vi "AutoWfmToSpreadsheet_2017.vi"() -> ()   [LabVIEW 2017]
uses:
  <vilib>/Waveform/WDTFileIO.llb/Read Waveform from File.vi
  <vilib>/Waveform/WDTFileIO.llb/Export Waveforms To Spreadsheet File (1D).vi
  <vilib>/Waveform/WDTOps.llb/WDT Index Channel DBL.vi
panel:
  out "?":string
  out "Sinal adquirido":waveform(dbl)(graph)
  in  "?":bool
  in  "Escolher arquivo":i32
  out "Sinal de Referência":waveform(dbl)(graph)
  in  "V para Exportar/ F para Visualizar":bool
  out "result string":string
  in  "Local da pasta com arquivos wfm":path=path "C:/Users/lucas/Documents/GitHub/INT/Novo Ensaio US/NOVOS_SINAIS/sinais/wfm"
  out "element":string
  out "Numeric":i32
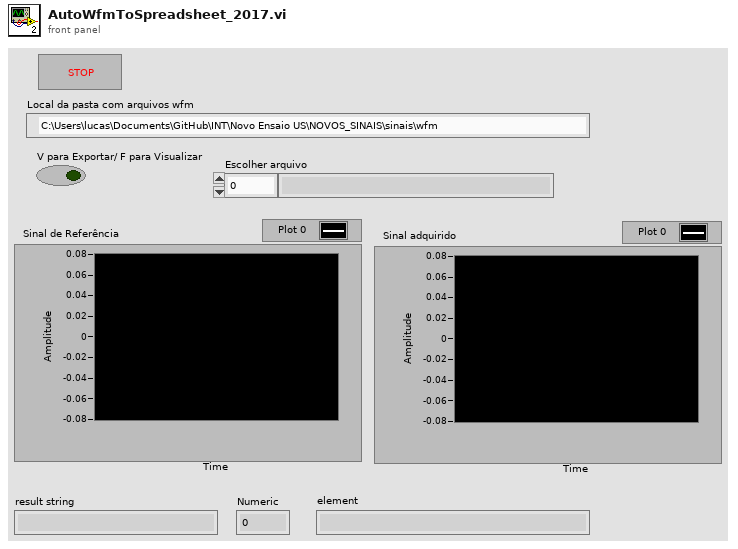
[diagram p1: front panel]
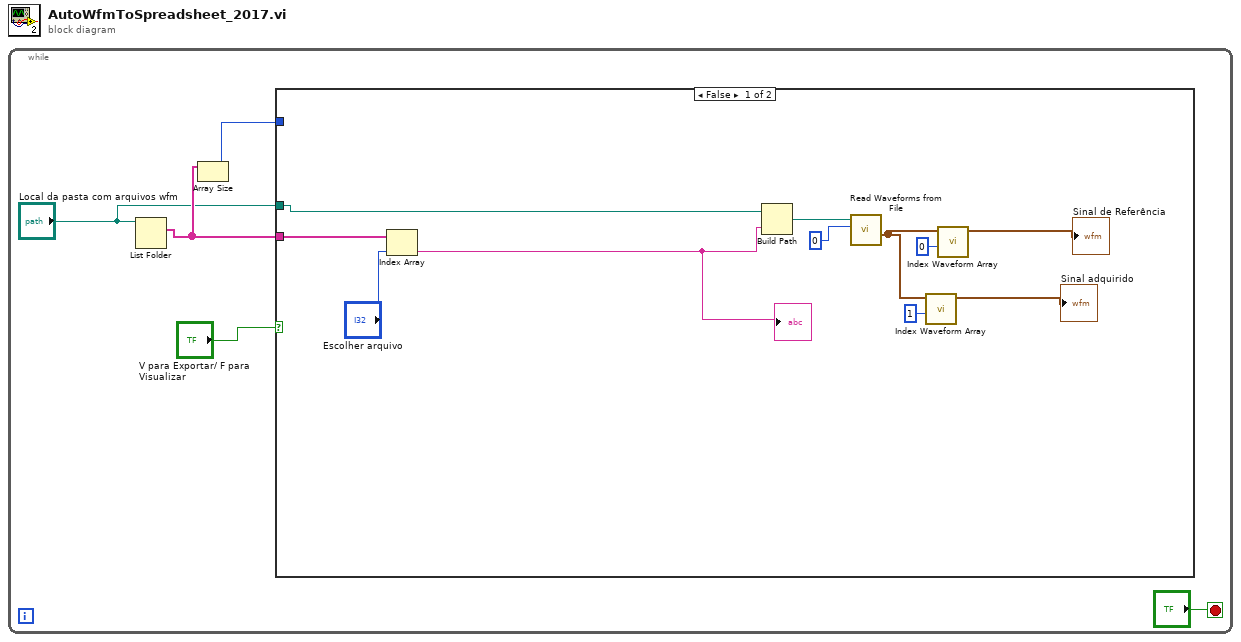
[diagram p0: block diagram]
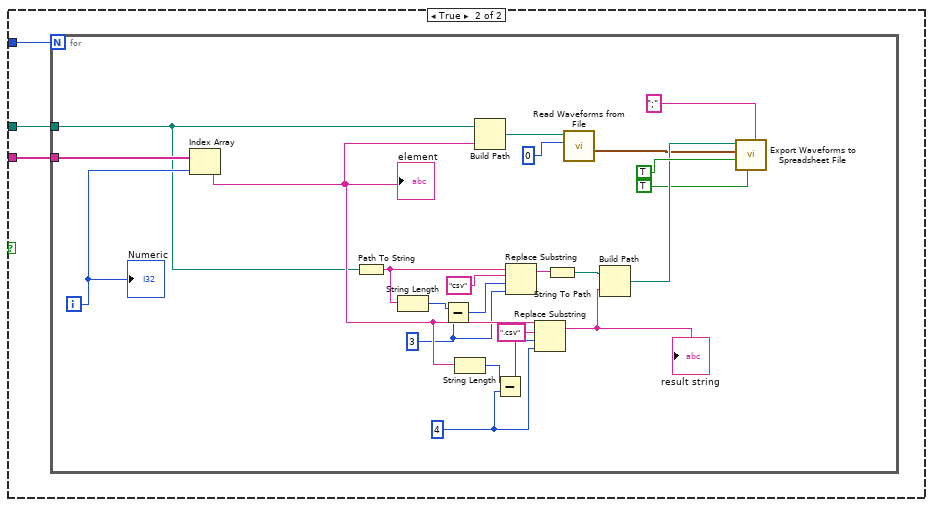
[diagram p2: hidden frame]
diagram:
  n1 = while {
    stop <- "?" stop-if-true
    n2 = List Folder(path="Local da pasta com arquivos wfm") -> (filenames=w5:string[])  [unwired: 3 in, 3 out]
    n3 = Array Size(array=w5) -> (size(s)=w4:i32)
    n4 = case shown="False" "V para Exportar/ F para Visualizar" {
      tunnel: w5 -> [w14 w19]
      tunnel: w4 -> [_ w18]
      tunnel: "Local da pasta com arquivos wfm" -> [w6 w17]
      frame False {
        n5 = Index Array(array=w14, index="Escolher arquivo") -> (element=w9:string)
        "?" <- w9
        n6 = Build Path(base path=w6, name or relative path=w9) -> (appended path=w16:path)
        n7 = call-poly <vilib>:"Read Waveforms from File.vi"("offset (records:0)"=0, "file path (dialog if empty)"=w16) -> ("all waveforms in record"=w10:waveform(dbl)[])  [unwired: 4 in, 3 out]
        n8 = call-poly <vilib>:"Index Waveform Array.vi"("index"=1, "waveform array"=w10) -> ("waveform"=→"Sinal adquirido":waveform(dbl))  [unwired: 8 in, 1 out]
        n9 = call-poly <vilib>:"Index Waveform Array.vi"("index"=0, "waveform array"=w10) -> ("waveform"=→"Sinal de Referência":waveform(dbl))  [unwired: 8 in, 1 out]
      }
      frame True {
        n10 = for {
          N: w18 -> [_]
          tunnel: w19 -> [w42]
          tunnel: w17 -> [w27]
          i -> [w41]
          w22 = 3 ("y")
          w31 = 4 ("length (len. of substring)")
          n11 = Index Array(array=w42, index=w41) -> (element=w32:string)
          "element" <- w32
          n12 = Path To String(path=w27) -> (string=w25:string)
          n13 = String Length(string=w25) -> (length=w24:i32)
          n14 = Subtract(x=w24, y=w22) -> (x-y=w23:i32)
          n15 = String Length(string=w32) -> (length=w30:i32)
          n16 = Build Path(base path=w27, name or relative path=w32) -> (appended path=w39:path)
          n17 = Subtract(x=w30, y=w31) -> (x-y=w29:i32)
          n18 = Replace Substring(2:w22, 3:w23, 4:"csv" ("substring (\"\")"), 5:w25) -> (1:w21:string)  [unwired: 1 out]
          n19 = Replace Substring(2:w31, 3:w29, 4:".csv" ("substring (\"\")"), 5:w32) -> (1:w33:string)  [unwired: 1 out]
          "result string" <- w33
          n20 = String To Path(string=w21) -> (path=w20:path)
          n21 = call-poly <vilib>:"Read Waveforms from File.vi"("offset (records:0)"=0, "file path (dialog if empty)"=w39) -> ("all waveforms in record"=w28:waveform(dbl)[])  [unwired: 4 in, 3 out]
          n22 = Build Path(base path=w20, name or relative path=w33) -> (appended path=w36:path)
          n23 = call-poly <vilib>:"Export Waveforms to Spreadsheet File.vi"("delimiter (Tab)"=";", "append to file? (new file:F)"=TRUE, "multiple time columns? (single:F)"=TRUE, "waveforms"=w28, "file path (dialog if empty)"=w36) -> ()  [unwired: 5 in, 2 out]
          "Numeric" <- w41
        }
      }
    }
  }
